vi "Qury table data.vi"(8 "error in (no error)":errorcluster caption="错误输入（无错误）", 9 "CMD":string, 10 "Tablename":string, 11 "Connncet State":T1) -> (0 "error out":errorcluster caption="错误输出", 1 "number of columns":i32, 2 "columns":string[](array[string]), 3 "data":string[][](array[string]))   [LabVIEW 2014]
uses:
  <vilib>/addons/database/NI_Database_API.lvlib
  <vilib>/addons/database/_DB Variant To Data/Database Variant To Data.xnode
  <vilib>/addons/database/Connection.llb/DB Tools Open Connec (String).vi
  Ctr/Constr.ctl
  <vilib>/addons/database/Connection.llb/Conn ObjectReference.ctl
  Ctr/Conneect State.ctl
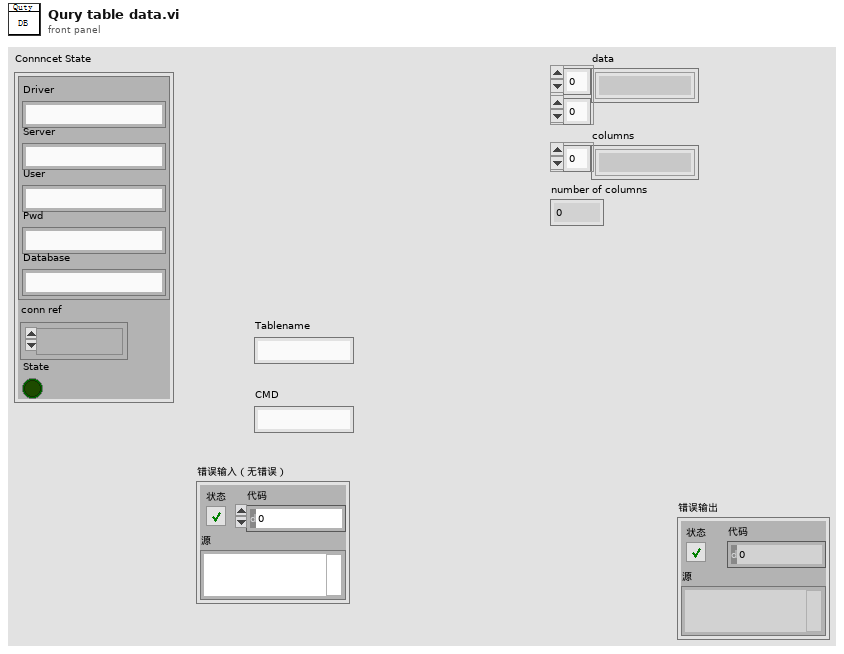
[diagram p1: front panel]
types:
  T1 = typedef "Conneect State.ctl" = cluster{"Constr":T2, "conn ref":T3, "State":bool}
  T2 = typedef "Constr.ctl" = cluster{"Driver":string, "Server":string, "User":string, "Pwd":string, "Database":string}
  T3 = typedef "NI_Database_API.lvlib/Conn ObjectReference.ctl" = refnum<k1>
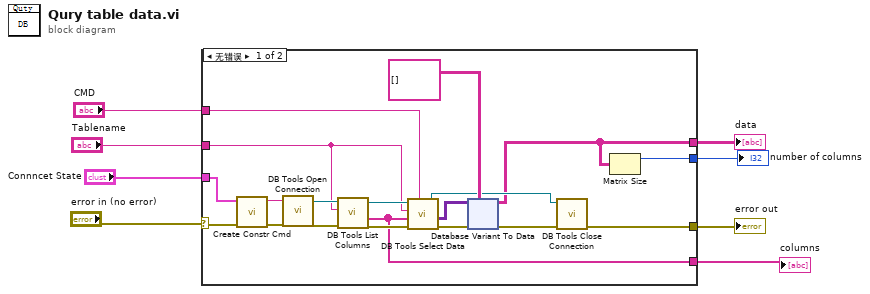
[diagram p0: block diagram]
diagram:
  n1 = case shown="无错误" "error in (no error)" {
    selector: "error in (no error)" -> [w12 w72]
    tunnel: "Tablename" -> [w22 _]
    tunnel: "CMD" -> [w23 _]
    tunnel: [w16 w72] -> w5
    tunnel: [w10 _] -> w4
    tunnel: [w15 _] -> w3
    tunnel: "Connncet State" -> [w11 _]
    tunnel: [w9 _] -> w1
    frame No Error {
      n2 = call "Create Constr Cmd.vi"("error in (no error)"=w12, "Connncet State"=w11) -> ("error out"=w14:errorcluster, "Constr"=w13:string)  [unwired: 8 in]
      n3 = call-poly <vilib>:"DB Tools Open Connection.vi"("error in (no error)"=w14, "connection information"=w13) -> ("error out"=w27:errorcluster, "connection reference"=w26:T3)  [unwired: 6 in]
      n4 = call <vilib>:"DB Tools List Columns.vi"("error in (no error)"=w27, "table"=w22, "connection reference"=w26) -> ("error out"=w25:errorcluster, "columns"=w15:string[], "connection reference out"=w24:T3)  [unwired: 1 in, 1 out]
      n5 = call <vilib>:"DB Tools Select Data.vi"("condition"=w23, "error in (no error)"=w25, "columns"=w15, "table"=w22, "connection reference"=w24) -> ("error out"=w21:errorcluster, "data"=w20:variant[][], "connection reference out"=w17:T3)  [unwired: 1 in]
      n6 = xnode "Database Variant To Data"("database variant"=w20, "error in (no error)"=w21, "type"=string[][] []) -> ("data"=w10:string[][], "error out"=w18:errorcluster)
      n7 = call <vilib>:"DB Tools Close Connection.vi"("error in (no error)"=w18, "connection reference"=w17) -> ("error out"=w16:errorcluster)  [unwired: 5 in]
      n8 = Matrix Size(0:w10) -> (1:w9:i32)  [unwired: 1 out]
    }
    frame Error {
    }
  }
  "error out" <- w5
  "data" <- w4
  "columns" <- w3
  "number of columns" <- w1
